vi "Constant - Serial Wait Time (ms).vi"() -> (3 "milliseconds to wait":u32=50)   [LabVIEW 2021]
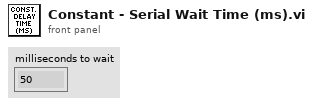
[diagram p1: front panel]
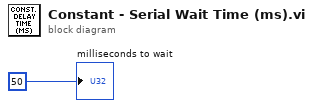
[diagram p0: block diagram]
diagram:
  "milliseconds to wait" <- u32 50 ("milliseconds to wait")
